vi "RCP_Speed_detection_Loop.vi"(0 "SI600.lvclass":refnum<class "SI600.lvclass">, 1 "Loop10":T4, 2 "Loop20":T3, 3 "Loop30":T2, 4 "Loop40":T1, 5 "error in (no error)":errorcluster) -> (14 "SI600.lvclass 2":refnum<class "SI600.lvclass">, 15 "RCP Speed Loop1":dbl, 16 "RCP Speed Loop2":dbl, 17 "RCP Speed Loop3":dbl, 18 "RCP Speed Loop4":dbl, 19 "error IO":errorcluster)   [LabVIEW 2022 SP3, in "SI600.lvclass"]
uses:
  SI600.lvclass
  SI600.lvclass/SI600.ctl
panel:
  # "SI600"
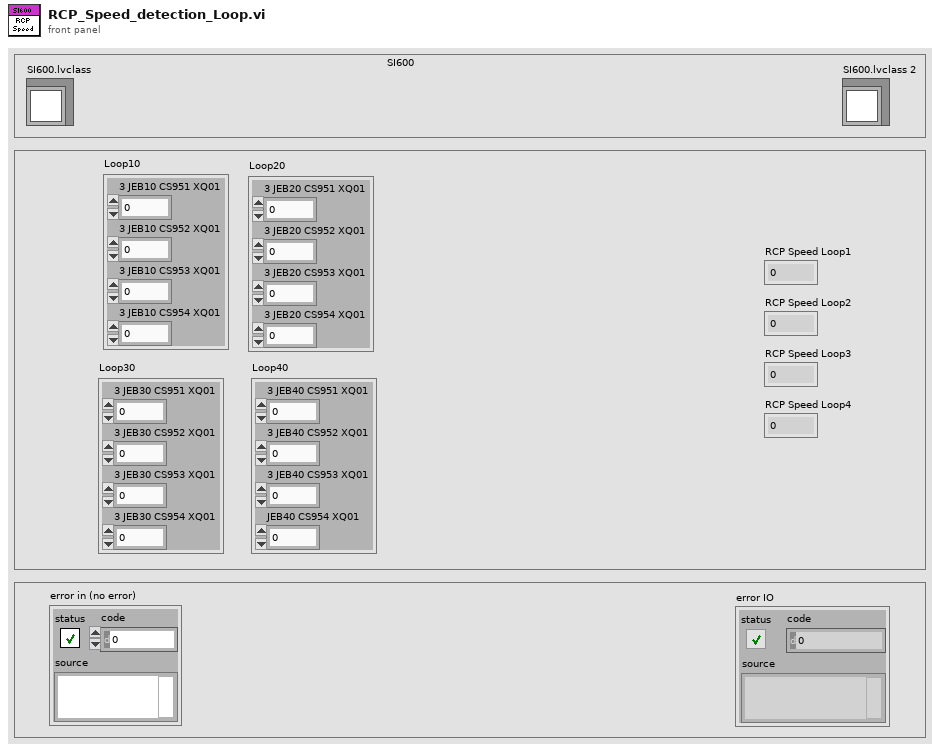
[diagram p1: front panel]
types:
  T1 = cluster{"3 JEB40 CS951 XQ01":dbl, "3 JEB40 CS952 XQ01":dbl, "3 JEB40 CS953 XQ01":dbl, "JEB40 CS954 XQ01":dbl}
  T2 = cluster{"3 JEB30 CS951 XQ01":dbl, "3 JEB30 CS952 XQ01":dbl, "3 JEB30 CS953 XQ01":dbl, "3 JEB30 CS954 XQ01":dbl}
  T3 = cluster{"3 JEB20 CS951 XQ01":dbl, "3 JEB20 CS952 XQ01":dbl, "3 JEB20 CS953 XQ01":dbl, "3 JEB20 CS954 XQ01":dbl}
  T4 = cluster{"3 JEB10 CS951 XQ01":dbl, "3 JEB10 CS952 XQ01":dbl, "3 JEB10 CS953 XQ01":dbl, "3 JEB10 CS954 XQ01":dbl}
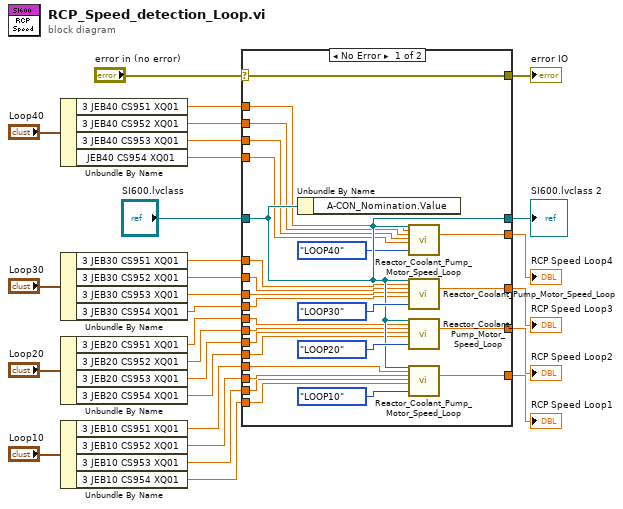
[diagram p0: block diagram]
diagram:
  n1 = Unbundle By Name("Loop40") -> ("3 JEB40 CS951 XQ01"=w4:dbl, "3 JEB40 CS952 XQ01"=w3:dbl, "3 JEB40 CS953 XQ01"=w2:dbl, "JEB40 CS954 XQ01"=w1:dbl)
  n2 = Unbundle By Name("Loop30") -> ("3 JEB30 CS951 XQ01"=w9:dbl, "3 JEB30 CS952 XQ01"=w8:dbl, "3 JEB30 CS953 XQ01"=w7:dbl, "3 JEB30 CS954 XQ01"=w6:dbl)
  n3 = Unbundle By Name("Loop20") -> ("3 JEB20 CS951 XQ01"=w14:dbl, "3 JEB20 CS952 XQ01"=w13:dbl, "3 JEB20 CS953 XQ01"=w12:dbl, "3 JEB20 CS954 XQ01"=w11:dbl)
  n4 = Unbundle By Name("Loop10") -> ("3 JEB10 CS951 XQ01"=w18:dbl, "3 JEB10 CS952 XQ01"=w17:dbl, "3 JEB10 CS953 XQ01"=w16:dbl, "3 JEB10 CS954 XQ01"=w15:dbl)
  n5 = case shown="No Error" "error in (no error)" {
    selector: "error in (no error)" -> [w51 w56]
    tunnel: "SI600.lvclass" -> [w50 w55]
    tunnel: [w51 w56] -> w26
    tunnel: [w50 w55] -> w25
    tunnel: [w49 _] -> w24
    tunnel: [w48 _] -> w23
    tunnel: [w47 _] -> w22
    tunnel: [w46 _] -> w21
    tunnel: w18 -> [w45 _]
    tunnel: w17 -> [w44 _]
    tunnel: w16 -> [w43 _]
    tunnel: w15 -> [w42 _]
    tunnel: w14 -> [w41 _]
    tunnel: w13 -> [w40 _]
    tunnel: w12 -> [w39 _]
    tunnel: w11 -> [w38 _]
    tunnel: w9 -> [w37 _]
    tunnel: w8 -> [w36 _]
    tunnel: w7 -> [w35 _]
    tunnel: w6 -> [w34 _]
    tunnel: w4 -> [w32 _]
    tunnel: w3 -> [w31 _]
    tunnel: w2 -> [w30 _]
    tunnel: w1 -> [w29 _]
    frame No Error {
      n6 = Unbundle By Name(w50) -> ()  [unwired: 1 out]
      n7 = call "Reactor_Coolant_Pump_Motor_Speed_Loop.vi"("SI600.lvclass in"=w50, "3 JEB CS951 XQ01"=w32, "3 JEB CS952 XQ01"=w31, "3 JEB CS953 XQ01"=w30, "3 JEB CS954 XQ01"=w29, "Loop"=enum16{"LOOP10", "LOOP20", "LOOP30", "LOOP40"}."LOOP40") -> ("3 JEB CS951"=w46:dbl)  [unwired: 15 in, 6 out]
      n8 = call "Reactor_Coolant_Pump_Motor_Speed_Loop.vi"("SI600.lvclass in"=w50, "3 JEB CS951 XQ01"=w37, "3 JEB CS952 XQ01"=w36, "3 JEB CS953 XQ01"=w35, "3 JEB CS954 XQ01"=w34, "Loop"=enum16{"LOOP10", "LOOP20", "LOOP30", "LOOP40"}."LOOP30") -> ("3 JEB CS951"=w47:dbl)  [unwired: 15 in, 6 out]
      n9 = call "Reactor_Coolant_Pump_Motor_Speed_Loop.vi"("SI600.lvclass in"=w50, "3 JEB CS951 XQ01"=w41, "3 JEB CS952 XQ01"=w40, "3 JEB CS953 XQ01"=w39, "3 JEB CS954 XQ01"=w38, "Loop"=enum16{"LOOP10", "LOOP20", "LOOP30", "LOOP40"}."LOOP20") -> ("3 JEB CS951"=w48:dbl)  [unwired: 15 in, 6 out]
      n10 = call "Reactor_Coolant_Pump_Motor_Speed_Loop.vi"("SI600.lvclass in"=w50, "3 JEB CS951 XQ01"=w45, "3 JEB CS952 XQ01"=w44, "3 JEB CS953 XQ01"=w43, "3 JEB CS954 XQ01"=w42, "Loop"=enum16{"LOOP10", "LOOP20", "LOOP30", "LOOP40"}."LOOP10") -> ("3 JEB CS951"=w49:dbl)  [unwired: 15 in, 6 out]
    }
    frame Error {
    }
  }
  "error IO" <- w26
  "SI600.lvclass 2" <- w25
  "RCP Speed Loop1" <- w24
  "RCP Speed Loop2" <- w23
  "RCP Speed Loop3" <- w22
  "RCP Speed Loop4" <- w21
